vi "test ActionVIOnCompile.vi"(8 "error in (no error)":errorcluster, 11 "TestCase in":refnum<class "SLSC Switch Unit Tests.lvclass">) -> (0 "error out":errorcluster, 3 "TestCase out":refnum<class "SLSC Switch Unit Tests.lvclass">)   [LabVIEW 2017, in "SLSC Switch Unit Tests.lvclass"]
uses:
  SLSC Switch Unit Tests.lvclass
  Scripting/Properties/SLSC Switch All Properties.ctl
  Shared/Compiled.Settings.ctl
  Shared/Communication Configuration.ctl
  Shared/Driver Configuration.ctl
  Shared/FIFO Indices.ctl
  Shared/Endpoint Configuration Cluster.ctl
  Shared/Endpoint Configuration Enum.ctl
  NationalInstruments.VeriStand.SystemDefinitionAPI
  Shared/Constants.vi
  <userlib>/_OpenG.lib/file/file.llb/Append Path to Root if Relative - Scalar__ogtk.vi
  <vilib>/NI Veristand/Custom Device API/Get Item Property (Variant).vi
  <vilib>/addons/_JKI Toolkits/VI Tester/TestCase.llb/TestCase.lvclass
  niveristand-custom-device-testing-tools/VeriStandTestUtilities/VeriStandTestUtilities.lvlib
  Scripting/SLSC Switch Scripting.lvlib
  System Explorer/SLSC Switch System Explorer.lvlib
  <vilib>/NI Veristand/Custom Device API/Custom Device API.lvlib
  Shared/SLSC Switch Shared.lvlib
  C:/Program Files (x86)/National Instruments/LabVIEW 2017/vi.lib/addons/_JKI Toolkits/VI Tester/TestCase.llb/TestCase.lvclass
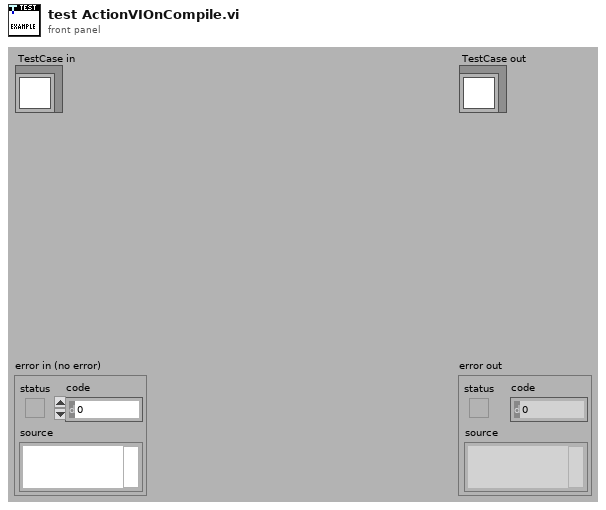
[diagram p1: front panel]
types:
  T1 = typedef "SLSC Switch Scripting.lvlib/SLSC Switch All Properties.ctl" = cluster{"Model":string, "Resource":string, "Topology":string, "Capabilities":string, "Description":string}
  T2 = typedef "SLSC Switch Shared.lvlib/Endpoint Configuration Cluster.ctl" = cluster{"Endpoint":string, "Configuration":T3}
  T3 = typedef "SLSC Switch Shared.lvlib/Endpoint Configuration Enum.ctl" = enum16{"Load", "Source", "Configuration"}
  T4 = typedef "SLSC Switch Shared.lvlib/Compiled.Settings.ctl" = cluster{"Custom Device Name":string, "Communication Configuration":T5, "Driver Configuration":T6, "FIFO Indices":T7}
  T5 = typedef "SLSC Switch Shared.lvlib/Communication Configuration.ctl" = cluster{"Consumer Queue Name":string}
  T6 = typedef "SLSC Switch Shared.lvlib/Driver Configuration.ctl" = cluster{"Resource Name":string, "Topology":string, "Switches JSON":string, "Source Channels":string[], "Configuration Channels":string[]}
  T7 = typedef "SLSC Switch Shared.lvlib/FIFO Indices.ctl" = cluster{"Status Channel":i32, "Heartbeat Channel":i32}
  T8 = typedef "Custom Device API.lvlib/Custom Device Item Ref.ctl" = u64
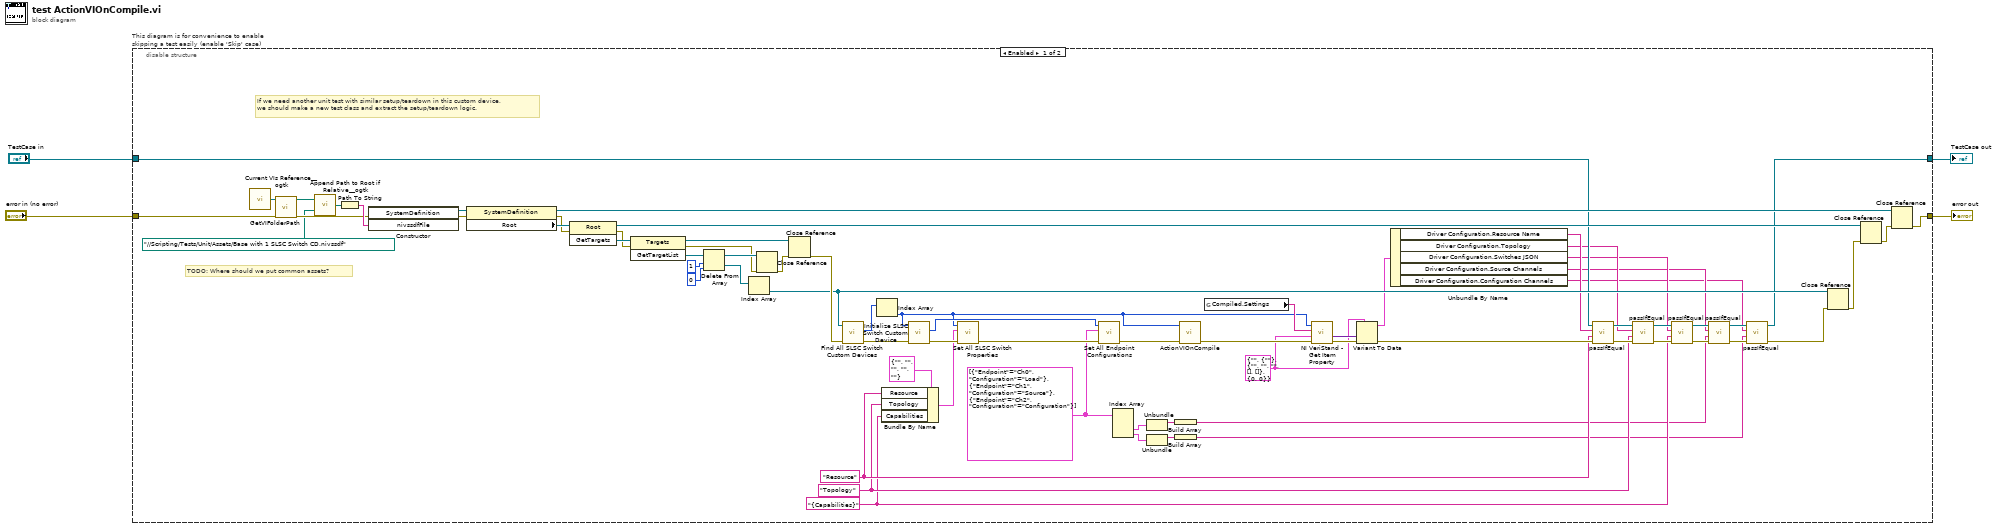
[diagram p0: block diagram]
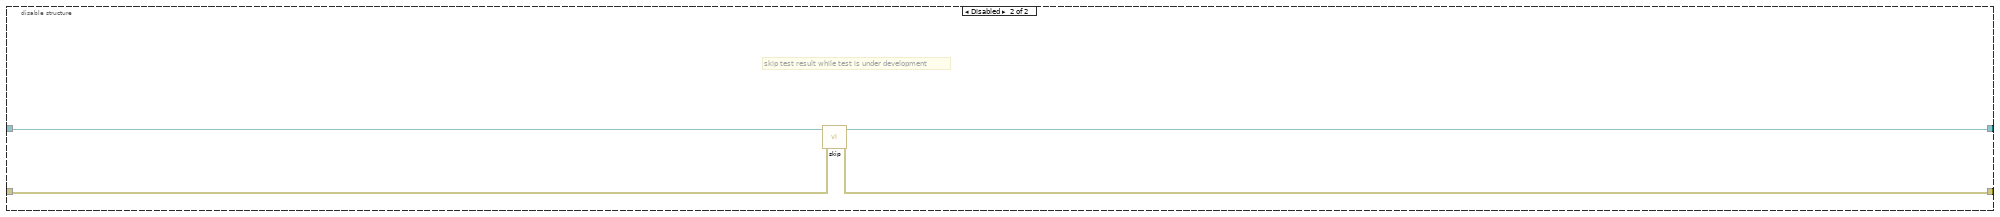
[diagram p2: hidden frame]
diagram:
  n1 = disable-structure "This diagram is for convenience to enable skipping a test easily (enable 'Skip' case)" shown="Enabled" {
    disable-tunnel: "TestCase in" -> [w32 w78]
    disable-tunnel: [w5 w76] -> w1
    disable-tunnel: [w53 w77] -> w3
    disable-tunnel: "error in (no error)" -> [w54 w75]
    frame Enabled {
      w19 = T2[] [{"Endpoint"="Ch0", "Configuration"=enum."Load"}, {"Endpoint"="Ch1", "Configuration"=enum."Source"}, {"Endpoint"="Ch2", "Configuration"=enum."Configuration"}] ("All Endpoint Configurations")
      w37 = T4 {"Custom Device Name"="", "Communication Configuration"={"Consumer Queue Name"=""}, "Driver Configuration"={"Resource Name"="", "Topology"="", "Switches JSON"="", "Source Channels"=[], "Configuration Channels"=[]}, "FIFO Indices"={"Status Channel"=0, "Heartbeat Channel"=0}} ("Compiled.Settings")
      w22 = "{Capabilities}" ("Capabilities")
      w26 = "Topology" ("Topology")
      w30 = "Resource" ("Resource")
      # "TODO: Where should we put common assets?"
      # "If we need another unit test with similar setup/teardown in this custom device,\nwe should make a new test class and extract the setup/teardown logic."
      n2 = call <userlib>:"Current VIs Reference__ogtk.vi"() -> ("Current VI's reference"=w58:refnum<vi>)  [unwired: 5 in]
      n3 = call "GetVIFolderPath.vi"("error in (no error)"=w54, "VI Reference in"=w58) -> ("error out"=w61:errorcluster, "VI Folder Path out"=w59:path)  [unwired: 8 in]
      n4 = call-poly <userlib>:"Append Path to Root if Relative__ogtk.vi"("Absolute or Relative Path"=path "../../Scripting/Tests/Unit/Assets/Base with 1 SLSC Switch CD.nivssdf", "Root Path"=w59) -> ("Absolute or Appended Path"=w60:path)
      n5 = Path To String(path=w60) -> (string=w63:string)
      n6 = constructor class="SystemDefinition"(error in=w61, "nivssdfFile"=w63) -> (reference out=w64:refnum<k24>, error out=w62:errorcluster)  [unwired: 2 in, 2 out]
      n7 = property class="SystemDefinition"(reference=w64, error in=w62) -> (reference out=w52:refnum<k24>, error out=w65:errorcluster, "Root"=w66:refnum<k24>)
      n8 = invoke class="Root" method="GetTargets"(reference=w66, error in=w65) -> (reference out=w50:refnum<k24>, error out=w67:errorcluster, "GetTargets"=w68:refnum<k24>)  [unwired: 1 in]
      n9 = invoke class="Targets" method="GetTargetList"(reference=w68, error in=w67) -> (reference out=w73:refnum<k24>, error out=w70:errorcluster, "GetTargetList"=w69:refnum<k24>[])  [unwired: 1 in]
      n10 = Delete From Array(array=w69, length=1, index=0) -> (deleted portion=w74:refnum<k24>[], array with subset deleted=w71:refnum<k24>[])
      n11 = Index Array(array=w74) -> (element=w45:refnum<k24>)  [unwired: 1 in]
      n12 = Close Reference(reference=w71, error in (no error)=w70) -> (error out=w72:errorcluster)
      n13 = Close Reference(reference=w73, error in (no error)=w72) -> (error out=w48:errorcluster)
      n14 = call "Find All SLSC Switch Custom Devices.vi"("error in (no error)"=w48, "Target in"=w45) -> ("error out"=w46:errorcluster, "SLSC Switch Custom Device Ref IDs"=w47:T8[])  [unwired: 7 in, 1 out]
      n15 = Index Array(array=w47) -> (element=w20:T8)  [unwired: 1 in]
      n16 = Bundle By Name(cluster=T1 {"Model"="", "Resource"="", "Topology"="", "Capabilities"="", "Description"=""} ("SLSC Switch All Properties"), "Resource"=w30, "Topology"=w26, "Capabilities"=w22) -> (w42:T1)
      n17 = call "Initialize SLSC Switch Custom Device.vi"("error in (no error)"=w46, "SLSC Switch Custom Device Ref in"=w20) -> ("error out"=w44:errorcluster, "Endpoint Configuration Section Ref"=w21:T8)  [unwired: 7 in, 1 out]
      n18 = call "Set All SLSC Switch Properties.vi"("error in (no error)"=w44, "SLSC Switch All Properties"=w42, "SLSC Switch Custom Device Ref in"=w20) -> ("error out"=w35:errorcluster)  [unwired: 7 in, 1 out]
      n19 = call "Set All Endpoint Configurations.vi"("error in (no error)"=w35, "All Endpoint Configurations"=w19, "Endpoint Configuration Section Ref in"=w21) -> ("error out"=w34:errorcluster)  [unwired: 7 in, 1 out]
      n20 = Index Array(array=w19) -> (element #2=w11:T2, element #3=w10:T2)  [unwired: 3 in, 1 out]
      n21 = Unbundle(w11) -> ("Endpoint"=w9:string)  [unwired: 1 out]
      n22 = Unbundle(w10) -> ("Endpoint"=w8:string)  [unwired: 1 out]
      n23 = Build Array(w9) -> (w7:string[])
      n24 = Build Array(w8) -> (w6:string[])
      n25 = call "ActionVIOnCompile.vi"("error in (no error)"=w34, "Device Item Ref in"=w20) -> ("error out"=w41:errorcluster)  [unwired: 9 in]
      n26 = global read "Constants.vi" "Compiled.Settings"() -> (w40:string)
      n27 = call-poly <vilib>:"NI VeriStand - Get Item Property.vi"("error in (no error)"=w41, "Default Value"=w37, "Property Name"=w40, "Item Ref in"=w20) -> ("error out"=w39:errorcluster, "Value"=w38:variant)  [unwired: 4 in, 2 out]
      n28 = Variant To Data(error in=w39, type=w37, Variant=w38) -> (data=w36:T4, error out=w33:errorcluster)
      n29 = Unbundle By Name(w36) -> ("Driver Configuration.Resource Name"=w31:string, "Driver Configuration.Topology"=w27:string, "Driver Configuration.Switches JSON"=w23:string, "Driver Configuration.Source Channels"=w16:string[], "Driver Configuration.Configuration Channels"=w13:string[])
      n30 = call-dynamic "passIfEqual.vi"("error in (no error)"=w33, "y"=w30, "x"=w31, "TestCase in"=w32) -> ("error out"=w28:errorcluster, "TestCase out"=w29:refnum<class "SLSC Switch Unit Tests.lvclass">)  [unwired: 6 in]
      n31 = call-dynamic "passIfEqual.vi"("error in (no error)"=w28, "y"=w26, "x"=w27, "TestCase in"=w29) -> ("error out"=w25:errorcluster, "TestCase out"=w24:refnum<class "SLSC Switch Unit Tests.lvclass">)  [unwired: 6 in]
      n32 = call-dynamic "passIfEqual.vi"("error in (no error)"=w25, "y"=w22, "x"=w23, "TestCase in"=w24) -> ("error out"=w17:errorcluster, "TestCase out"=w18:refnum<class "SLSC Switch Unit Tests.lvclass">)  [unwired: 6 in]
      n33 = call-dynamic "passIfEqual.vi"("error in (no error)"=w17, "y"=w7, "x"=w16, "TestCase in"=w18) -> ("error out"=w14:errorcluster, "TestCase out"=w15:refnum<class "SLSC Switch Unit Tests.lvclass">)  [unwired: 6 in]
      n34 = call-dynamic "passIfEqual.vi"("error in (no error)"=w14, "y"=w6, "x"=w13, "TestCase in"=w15) -> ("error out"=w12:errorcluster, "TestCase out"=w5:refnum<class "SLSC Switch Unit Tests.lvclass">)  [unwired: 6 in]
      n35 = Close Reference(reference=w45, error in (no error)=w12) -> (error out=w49:errorcluster)
      n36 = Close Reference(reference=w50, error in (no error)=w49) -> (error out=w51:errorcluster)
      n37 = Close Reference(reference=w52, error in (no error)=w51) -> (error out=w53:errorcluster)
    }
    frame Disabled {
      # "skip test result while test is under development"
      n38 = call <vilib>:"skip.vi"("error in (no error)"=w75, "TestCase in"=w78) -> ("error out"=w77:errorcluster, "TestCase out"=w76:refnum<class "SLSC Switch Unit Tests.lvclass">)  [unwired: 8 in]
    }
  }
  "error out" <- w3
  "TestCase out" <- w1
